vi "_API_BINANCE_DELETE_CanelOrder.vi"(0 "BinanceAPI in":refnum<class "BinanceAPI_.lvclass">, 5 "NewOrder_PARAMS":T1={"symbol (eg. BTCUSDT)"="CAKEUSDT", "OrderId"=0, "recvWindow"=5000, "timestamp"=0, "origClientOrderID"="NaN", "newClientOrderID"="NaN"}, 11 "error in (no error)":errorcluster) -> (4 "BinanceAPI out":refnum<class "BinanceAPI_.lvclass">, 14 "Body":string, 15 "error out":errorcluster)   [LabVIEW 2022 SP3, in "BinanceAPI_.lvclass"]
doc: "Cancel an active order."
uses:
  BinanceAPI_.lvclass
  BinanceAPI_.lvclass/BinanceAPI_.ctl
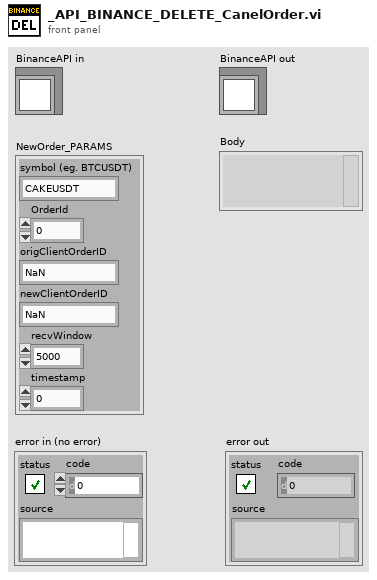
[diagram p1: front panel]
types:
  T1 = cluster{"symbol (eg. BTCUSDT)":string, "OrderId":i32, "recvWindow":i32, "timestamp":i32, "origClientOrderID":string, "newClientOrderID":string}
  T2 = enum16{"SPOT", "USDT_FUTURES", "COIN_FUTURES", "VANILLA"}
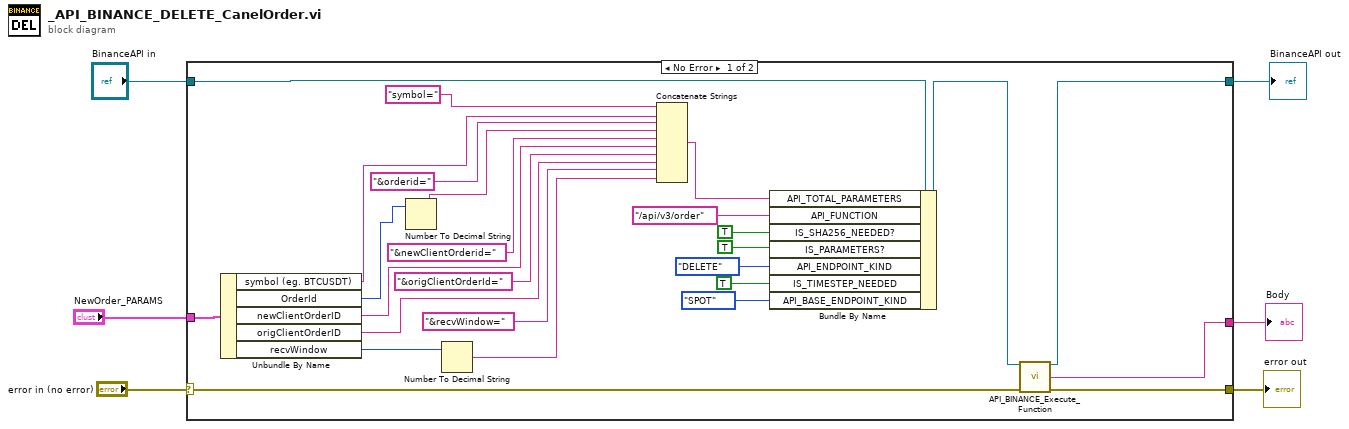
[diagram p0: block diagram]
diagram:
  n1 = case shown="No Error" "error in (no error)" {
    selector: "error in (no error)" -> [w10 w34]
    tunnel: [w9 w34] -> w5
    tunnel: [w11 w33] -> w2
    tunnel: "BinanceAPI in" -> [w26 w33]
    tunnel: "NewOrder_PARAMS" -> [w29 _]
    tunnel: [w7 _] -> w1
    frame No Error {
      n2 = Unbundle By Name(w29) -> ("symbol (eg. BTCUSDT)"=w14:string, "OrderId"=w17:i32, "newClientOrderID"=w23:string, "origClientOrderID"=w21:string, "recvWindow"=w18:i32)
      n3 = Number To Decimal String(number=w17) -> (decimal integer string=w16:string)  [unwired: 1 in]
      n4 = Number To Decimal String(number=w18) -> (decimal integer string=w19:string)  [unwired: 1 in]
      n5 = Concatenate Strings("symbol=" ("Symbol"), w14, "&orderid=" ("Symbol"), w16, "&newClientOrderid=" ("Symbol"), w23, "&origClientOrderId=" ("Symbol"), w21, "&recvWindow=" ("Symbol"), w19) -> (w28:string)
      n6 = Bundle By Name(cluster=w26, "API_TOTAL_PARAMETERS"=w28, "API_FUNCTION"="/api/v3/order", "IS_SHA256_NEEDED?"=TRUE, "IS_PARAMETERS?"=TRUE, "API_ENDPOINT_KIND"=enum16{"POST", "DELETE", "GET", "PUT"}."DELETE", "IS_TIMESTEP_NEEDED"=TRUE ("IS_PARAMETERS?"), "API_BASE_ENDPOINT_KIND"=T2."SPOT") -> (w12:refnum<class "BinanceAPI_.lvclass">)
      n7 = call "API_BINANCE_Execute_Function.vi"("BinanceAPI in"=w12, "error in (no error)"=w10) -> ("BinanceAPI out"=w11:refnum<class "BinanceAPI_.lvclass">, "Body"=w7:string, "error out"=w9:errorcluster)  [unwired: 9 in, 2 out]
    }
    frame Error {
    }
  }
  "error out" <- w5
  "BinanceAPI out" <- w2
  "Body" <- w1
